vi "Actor Core.vi"(8 "error in":errorcluster, 11 "Transfer Beginner in":refnum<class "Transfer Beginner.lvclass">) -> (0 "error out":errorcluster, 3 "Actor out":refnum<class "Actor.lvclass">)   [LabVIEW 2020, in "CANopen.lvlib" / "SDO Manager.lvlib" / "Transfer Beginner.lvlib" / "Transfer Beginner.lvclass"]
doc: "<p>(<strong>Filename</strong>: <span class=\"dnl\">Actor Framework.lvlib:Actor.lvclass:Actor Core.vi</span>)</p>\n<p>Receives messages to the actor, reacts to them, and initiates any error handling that may shut the actor down.</p>\n<p>Descendant classes may override this VI to append parallel tasks for the actor to complete while it handles messages. Overrides use the <a href=\"nihelplauncher://docs/csh?context=lvcore_glang_udclass\">Call Parent Class Method</a> node.</p>"
uses:
  Transfer Beginner.lvclass
  C:/Program Files/National Instruments/LabVIEW 2026/vi.lib/ActorFramework/Actor/Actor.lvclass
  <vilib>/ActorFramework/Actor/Actor.lvclass
  SDO Transfer/SDO Transfer.lvclass
  <vilib>/ActorFramework/Actor/Actor.lvclass/Actor.ctl
  <vilib>/ActorFramework/Message Enqueuer/Message Enqueuer.lvclass/Message Enqueuer.ctl
  Transfer Beginner.lvclass/Transfer Beginner.ctl
  SDO Transfer/SDO Transfer.lvclass/SDO Transfer.ctl
  <vilib>/ActorFramework/Stop Msg/Stop Msg.lvclass
  C:/Program Files/National Instruments/LabVIEW 2026/vi.lib/ActorFramework/Message/Message.lvclass
  <vilib>/ActorFramework/Message Enqueuer/Message Enqueuer.lvclass
  SDO Transfer/SDO abort code.ctl
  Typedefs/SDO Result.ctl
  SDO Transfer/SDO Transfer Result.ctl
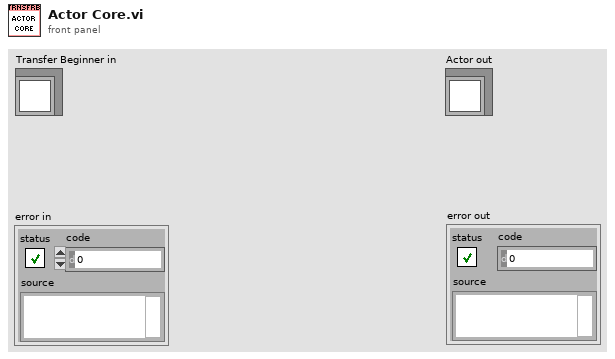
[diagram p1: front panel]
types:
  T1 = typedef "CANopen.lvlib/SDO Manager.lvlib/SDO Transfer.lvclass/SDO Transfer Result.ctl" = cluster{"SDO Result":T2, "Error":errorcluster}
  T2 = typedef "CANopen.lvlib/SDO Manager.lvlib/SDO Transfer.lvclass/SDO Result.ctl" = cluster{"Success":bool, "SDO abort code":cluster{"Null":bool, "Value":T3}, "Data":cluster{"Null":bool, "Data":u8[]}}
  T3 = typedef "CANopen.lvlib/SDO Manager.lvlib/SDO Transfer.lvclass/SDO abort code.ctl" = u32
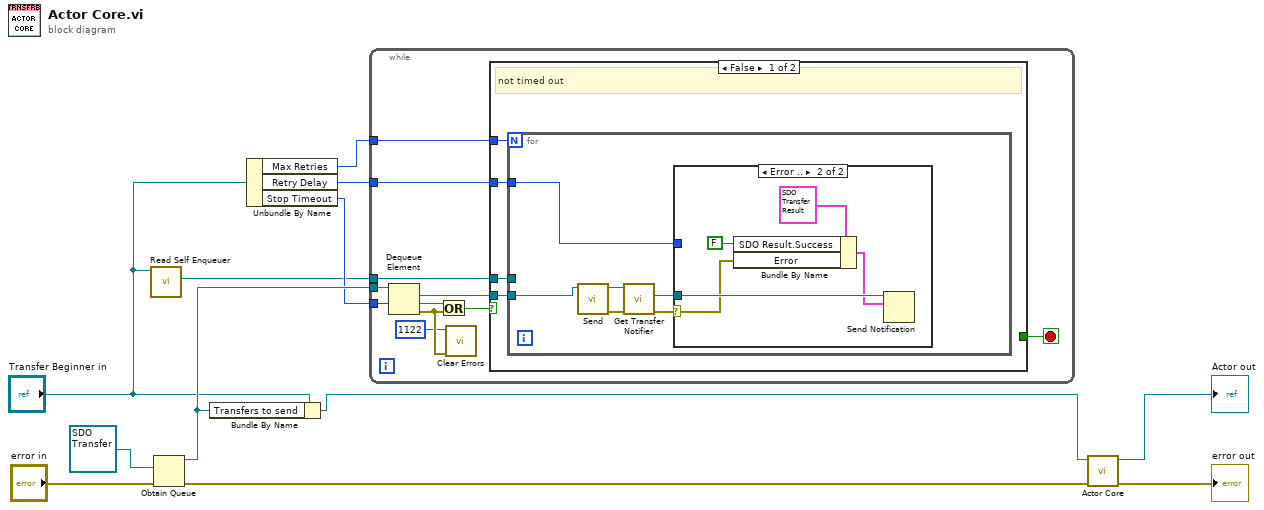
[diagram p0: block diagram]
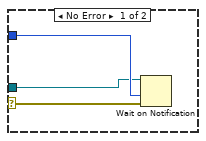
[diagram p2: hidden frame]
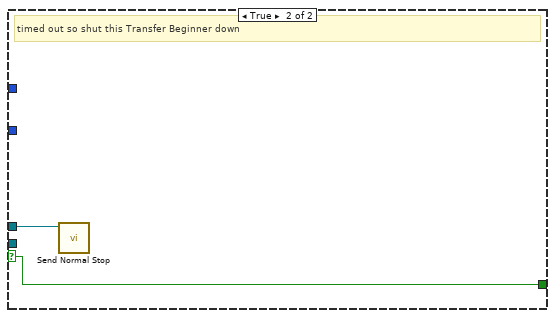
[diagram p3: hidden frame]
diagram:
  n1 = call <vilib>:"Read Self Enqueuer.vi"("Actor"="Transfer Beginner in") -> ("Self Enqueuer"=w1:refnum<class "Message Enqueuer.lvclass">)  [unwired: 10 in]
  n2 = Obtain Queue(element data type=refnum<class "SDO Transfer.lvclass"> refnum ("SDO Transfer"), error in (no error)="error in") -> (queue out=w6:refnum<queue>, error out=w9:errorcluster)  [unwired: 3 in, 1 out]
  n3 = Bundle By Name(cluster="Transfer Beginner in", "Transfers to send"=w6) -> (w7:refnum<class "Transfer Beginner.lvclass">)
  n4 = Unbundle By Name("Transfer Beginner in") -> ("Max Retries"=w5:u8, "Retry Delay"=w4:i32, "Stop Timeout"=w3:i32)
  n5 = while {
    tunnel: w6 -> [w23]
    tunnel: w5 -> [w21]
    tunnel: w4 -> [w20]
    tunnel: w3 -> [w19]
    tunnel: w1 -> [w17]
    stop <- w15 stop-if-true
    n6 = Dequeue Element(queue=w23, timeout in ms (-1)=w19) -> (element=w22:refnum<class "SDO Transfer.lvclass">, timed out?=w18:bool, error out=w14:errorcluster)  [unwired: 1 in, 1 out]
    n7 = Or(x=w18, y=w14) -> (x .or. y?=w16:bool)
    n8 = call <vilib>:"Clear Errors.vi"("error in (no error)"=w14, "specific error code to clear (0: all)"=1122) -> ()  [unwired: 4 in, 2 out]
    n9 = case shown="False" w16 {
      selector: w16 -> [_ w42]
      tunnel: w22 -> [w27 _]
      tunnel: w21 -> [w26 _]
      tunnel: w20 -> [w25 _]
      tunnel: w17 -> [w24 w43]
      tunnel: [_ w42] -> w15
      frame False {
        # "not timed out"
        n10 = for {
          N: w26 -> [_]
          tunnel: w27 -> [w33]
          tunnel: w25 -> [w32]
          tunnel: w24 -> [_]
          n11 = call-dynamic "Send.vi"("SDO Transfer in"=w33) -> ("error out"=w31:errorcluster, "SDO Transfer out"=w30:refnum<class "SDO Transfer.lvclass">)  [unwired: 9 in]
          n12 = call "Get Transfer Notifier.vi"("error in"=w31, "SDO Transfer in"=w30) -> ("error out"=w29:errorcluster, "SDO Transfer Notifier"=w28:refnum<notifier>)  [unwired: 7 in, 1 out]
          n13 = case shown="Error .." w29 {
            selector: w29 -> [w35 w37]
            tunnel: w28 -> [w34 w41]
            tunnel: w32 -> [w36 _]
            frame No Error {
              n14 = Wait on Notification(notifier=w34, timeout in ms (-1)=w36, error in (no error)=w35) -> ()  [unwired: 1 in, 4 out]
            }
            frame Error {
              n15 = Bundle By Name(cluster=T1 {"SDO Result"={"Success"=FALSE, "SDO abort code"={"Null"=FALSE, "Value"=0}, "Data"={"Null"=FALSE, "Data"=[]}}, "Error"={"status"=TRUE, "code"=84082688, "source"=""}} ("notification"), "SDO Result.Success"=FALSE ("Success"), "Error"=w37) -> (w39:T1)
              n16 = Send Notification(notification=w39, notifier=w41) -> ()  [unwired: 1 in, 2 out]
            }
          }
        }
      }
      frame True {
        # "timed out so shut this Transfer Beginner down"
        n17 = call <vilib>:"Send Normal Stop.vi"("Message Enqueuer"=w43) -> ()  [unwired: 10 in, 1 out]
      }
    }
  }
  n18 = call-parent "Actor Core.vi"("error in"=w9, "Actor in"=w7) -> ("error out"=→"error out":errorcluster, "Actor out"=→"Actor out":refnum<class "Actor.lvclass">)  [unwired: 8 in]
